vi "DLU with 4 Wire Handshake.vi"(6 "ready for output":bool=TRUE, 9 "Input Valid":bool=TRUE, 10 "Input Data":T3, 11 "Private Data In":T2={"DLU To SPI Engine Data FIFO"="DLU To SPI Engine Data", "SPI Engine to DLU Data FIFO"="SPI Engine to DLU Data", "Data to SPI Engine (Cache) Register"="Data to SPI Engine (Cache)", "SPI PHY Settings to SPI Engine (Cahche) Register"="SPI PHY Settings to SPI Engine (Cache)"}) -> (1 "Output Valid":bool=TRUE, 2 "Output Data":T1, 4 "ready for Input":bool)   [LabVIEW 2014, in "IO Node Logic Template_SPIBus0.lvlib"]
uses:
  IO Node Logic Template_SPIBus0.lvlib
  IONode/Node/Controls/Node_Command_Sent.ctl
  <vilib>/SPI API/SPIAPI/Controls/Internal Data (SPI API).ctl
  <vilib>/SPI API/SPIAPI/Controls/SPI Response Information.ctl
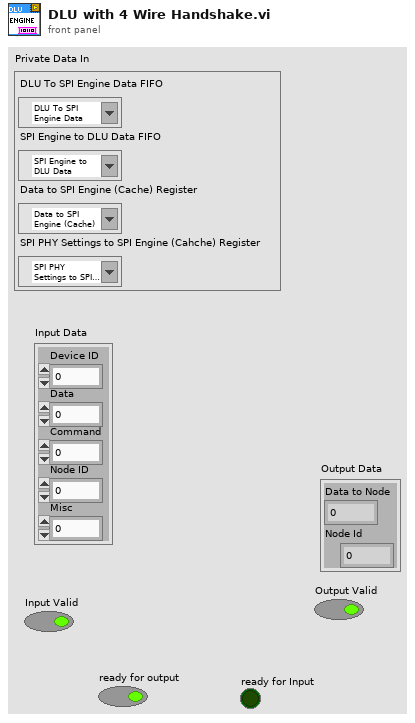
[diagram p1: front panel]
types:
  T1 = typedef "SPI Response Information.ctl" = cluster{"Data to Node":u64, "Node Id":u16}
  T2 = typedef "Internal Data (SPI API).ctl" = cluster{"DLU To SPI Engine Data FIFO":refnum<k21>, "SPI Engine to DLU Data FIFO":refnum<k21>, "Data to SPI Engine (Cache) Register":refnum<k21>, "SPI PHY Settings to SPI Engine (Cahche) Register":refnum<k21>}
  T3 = typedef "Node_Command_Sent.ctl" = cluster{"Device ID":u8, "Data":u64, "Command":u8, "Node ID":u8, "Misc":u8}
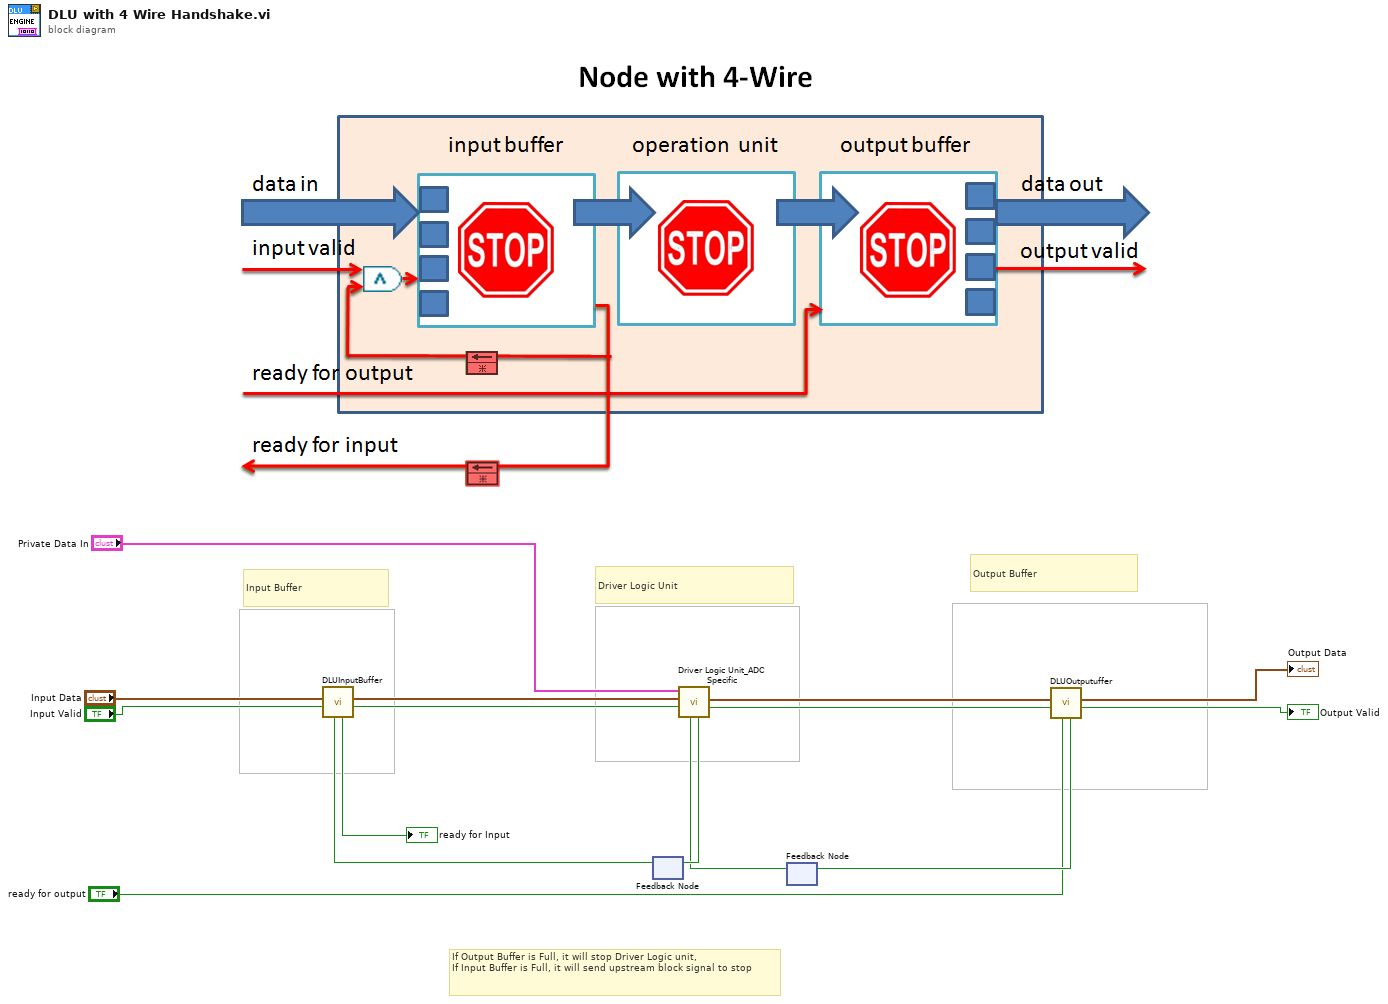
[diagram p0: block diagram]
diagram:
  # "If Output Buffer is Full, it will stop Driver Logic unit,\nIf Input Buffer is Full, it will send upstream block signal to stop"
  # "Input Buffer"
  # "Output Buffer"
  # "Driver Logic Unit"
  n1 = feedback #1() -> (w4:bool)  [unwired: 1 in]
  n2 = call "DLUInputBuffer.vi"("Ready for Output"=w4, "Input Valid"="Input Valid", "Input Data"="Input Data") -> (1:"Output Data"=w10:bool, 2:"Output Data"=w14:T3, "Ready For Input"=→"ready for Input":bool)  [unwired: 6 in]
  n3 = feedback #2() -> (w6:bool)  [unwired: 1 in]
  n4 = call "Driver Logic Unit_ADC Specific.vi"("Ready for Output"=w6, "New Cmd Valid?"=w10, "Command sent by Node"=w14, "Private Data In"="Private Data In") -> ("SPI Data Valid?"=w9:bool, "SPI Bus Read Data"=w2:T1, "Ready For Input?"=w15:bool)  [unwired: 4 in, 1 out]
  n5 = feedback-in #1(w15) -> ()
  n6 = call "DLUOutputuffer.vi"("Ready for Output"="ready for output", "Input Valid"=w9, "Input Data"=w2) -> ("Output Valid"=→"Output Valid":bool, "Output Data"=→"Output Data":cluster{"Data to Node":u64, "Node Id":u16}, "Ready For Input"=w8:bool)  [unwired: 6 in]
  n7 = feedback-in #2(w8) -> ()
